vi "Separate ROI.vi"(4 "Axis":bool, 7 "ROI Descriptor":T1 {"Contours"."Type" items=["No Selection", "Point", "Line", "Rectangle", "Oval", "Polygon", "Free", "Annulus", "Unused2", "Unused3", "Broken Line", "Free Hand Line", "Rotated Rectangle"]}) -> (2 "Right/Bottom ROI":T1 {"Contours"."Type" items=["No Selection", "Point", "Line", "Rectangle", "Oval", "Polygon", "Free", "Annulus", "Unused2", "Unused3", "Broken Line", "Free Hand Line", "Rotated Rectangle"]}, 3 "Left/Top ROI":T1 {"Contours"."Type" items=["No Selection", "Point", "Line", "Rectangle", "Oval", "Polygon", "Free", "Annulus", "Unused2", "Unused3", "Broken Line", "Free Hand Line", "Rotated Rectangle"]})   [LabVIEW 2020]
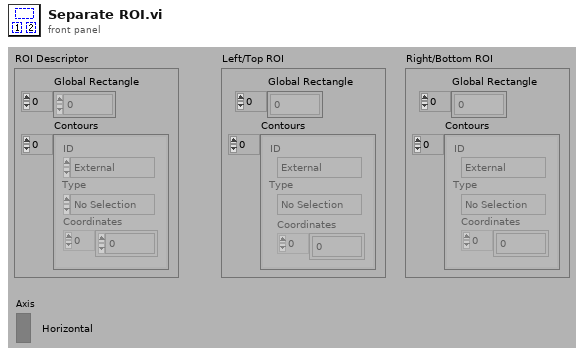
[diagram p1: front panel]
types:
  T1 = cluster{"Global Rectangle":i32[], "Contours":cluster{"ID":enum32{"External", "Internal"}, "Type":u32, "Coordinates":i32[]}[]}
  T2 = enum32{"No Selection", "Point", "Line", "Rectangle", "Oval", "Polygon", "Free", "Unused1", "Unused2", "Unused3", "Broken Line", "Free Hand Line"}
  T3 = cluster{"ID":enum32{"External", "Internal"}, "Type":u32, "Coordinates":i32[]}[]
  T4 = cluster{"ID":enum32{"External", "Internal"}, "Type":u32, "Coordinates":i32[]}
  T5 = cluster{"[0]":cluster{i32, i32}, "[1]":cluster{i32, i32}, "[2]":cluster{i32, i32}, "[3]":cluster{i32, i32}, "[4]":cluster{i32, i32}}
  T6 = cluster{"ID":enum32{"External", "Internal"}, "Type":enum32{"No Selection", "Point", "Line", "Rectangle", "Oval", "Polygon", "Free", "Unused1", "Unused2", "Unused3", "Broken Line", "Free Hand Line"}, dbl[]}
  T7 = cluster{"ID":enum32{"External", "Internal"}, "Type":enum32{"No Selection", "Point", "Line", "Rectangle", "Oval", "Polygon", "Free", "Unused1", "Unused2", "Unused3", "Broken Line", "Free Hand Line"}, dbl[]}[]
  T8 = cluster{"Global Rectangle":i32[], cluster{"ID":enum32{"External", "Internal"}, "Type":enum32{"No Selection", "Point", "Line", "Rectangle", "Oval", "Polygon", "Free", "Unused1", "Unused2", "Unused3", "Broken Line", "Free Hand Line"}, dbl[]}[]}
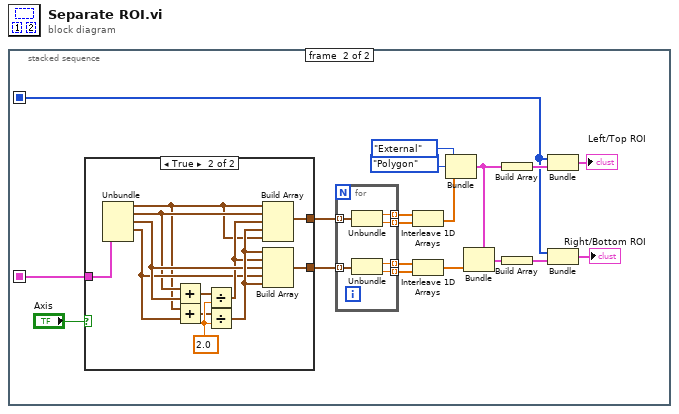
[diagram p0: block diagram]
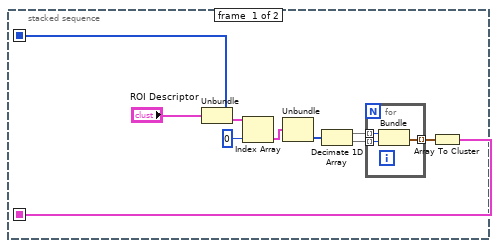
[diagram p2: hidden frame]
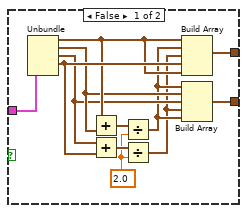
[diagram p3: hidden frame]
diagram:
  n1 = stacked-sequence {
    seq-local: [w2 _] -> [_ w16]
    seq-local: [w1 _] -> [_ w15]
    frame #0 {
      n2 = Unbundle("ROI Descriptor") -> ("Global Rectangle"=w2:i32[], "Contours"=w4:T3)
      n3 = Index Array(array=w4, index=0 ("Index")) -> (element=w6:T4)
      n4 = Unbundle(w6) -> ("Coordinates"=w7:i32[])  [unwired: 2 out]
      n5 = Decimate 1D Array(w7) -> (w8:i32[], w9:i32[])
      n6 = for {
        tunnel: w8 -> [w13] mode=indexing
        tunnel: w9 -> [w12] mode=indexing
        tunnel: [w11] -> w10 mode=indexing
        n7 = Bundle(w13, w12) -> (w11:cluster{i32, i32})  [unwired: 1 out]
      }
      n8 = Array To Cluster(array=w10) -> (cluster=w1:T5)
    }
    frame #1 {
      n9 = case shown="True" "Axis" {
        tunnel: [w44 w48] -> w30
        tunnel: [w43 w49] -> w29
        tunnel: w15 -> [w38 w50]
        frame False {
          w35 = 2.0 ("Index")
          n10 = Unbundle(w38) -> ("[0]"=w41:cluster{i32, i32}, "[1]"=w40:cluster{i32, i32}, "[2]"=w39:cluster{i32, i32}, "[3]"=w42:cluster{i32, i32})  [unwired: 1 out]
          n11 = Add(x=w41, y=w40) -> (x+y=w37:cluster{i32, i32})
          n12 = Add(x=w39, y=w42) -> (x+y=w36:cluster{i32, i32})
          n13 = Divide(x=w37, y=w35) -> (x/y=w34:cluster{dbl, dbl})
          n14 = Divide(x=w36, y=w35) -> (x/y=w33:cluster{dbl, dbl})
          n15 = Build Array(w41, w34, w33, w42, w41) -> (w43:cluster{dbl, dbl}[])
          n16 = Build Array(w34, w40, w39, w33, w34) -> (w44:cluster{dbl, dbl}[])
        }
        frame True {
          w53 = 2.0 ("Index")
          n17 = Unbundle(w50) -> ("[0]"=w45:cluster{i32, i32}, "[1]"=w46:cluster{i32, i32}, "[2]"=w55:cluster{i32, i32}, "[3]"=w47:cluster{i32, i32})  [unwired: 1 out]
          n18 = Add(x=w46, y=w55) -> (x+y=w51:cluster{i32, i32})
          n19 = Add(x=w45, y=w47) -> (x+y=w52:cluster{i32, i32})
          n20 = Divide(x=w51, y=w53) -> (x/y=w54:cluster{dbl, dbl})
          n21 = Divide(x=w52, y=w53) -> (x/y=w56:cluster{dbl, dbl})
          n22 = Build Array(w45, w46, w54, w56, w45) -> (w49:cluster{dbl, dbl}[])
          n23 = Build Array(w56, w54, w55, w47, w56) -> (w48:cluster{dbl, dbl}[])
        }
      }
      n24 = for {
        tunnel: w29 -> [w62] mode=indexing
        tunnel: [w61] -> w28 mode=indexing
        tunnel: [w60] -> w27 mode=indexing
        tunnel: w30 -> [w59] mode=indexing
        tunnel: [w58] -> w31 mode=indexing
        tunnel: [w57] -> w32 mode=indexing
        n25 = Unbundle(w62) -> (w61:dbl, w60:dbl)
        n26 = Unbundle(w59) -> (w58:dbl, w57:dbl)
      }
      n27 = Interleave 1D Arrays(w28, w27) -> (w22:dbl[])
      n28 = Interleave 1D Arrays(w31, w32) -> (w19:dbl[])
      n29 = Bundle("ID"=enum32{"External", "Internal"}."External", "Type"=T2."Polygon", w22) -> (w25:T6)  [unwired: 1 out]
      n30 = Bundle(cluster=w25, w19) -> (w21:T6)  [unwired: 2 out]
      n31 = Build Array(w25) -> (w26:T7)
      n32 = Build Array(w21) -> (w20:T7)
      n33 = Bundle("Global Rectangle"=w16, w26) -> (→"Left/Top ROI":T8)  [unwired: 1 out]
      n34 = Bundle("Global Rectangle"=w16, w20) -> (→"Right/Bottom ROI":T8)  [unwired: 1 out]
    }
  }
